vi "Timed_Display.vi"(2 "Message":string, 3 "Seconds to wait":dbl=1.0 format="%.2f") -> (0 "Stopped":bool)   [LabVIEW 2010]
doc: "Waits the number of seconds specified by the Seconds to Wait input, divided by the time dilation factor, if used."
panel:
  in  "stop":bool
  out "Seconds waited":u32(slide) scale=0.0..5.0
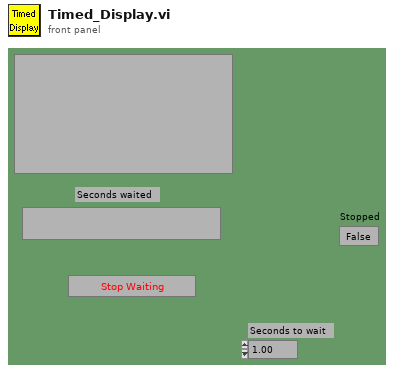
[diagram p1: front panel]
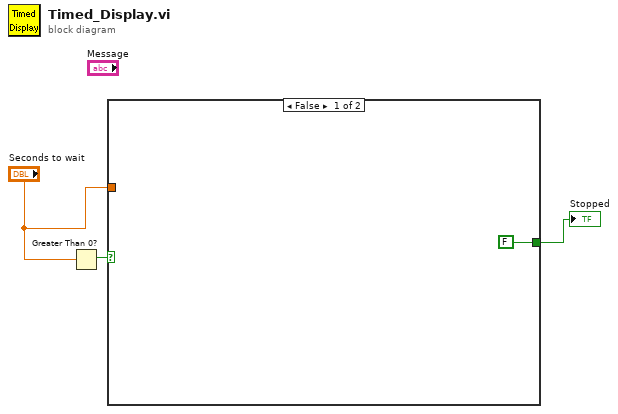
[diagram p0: block diagram]
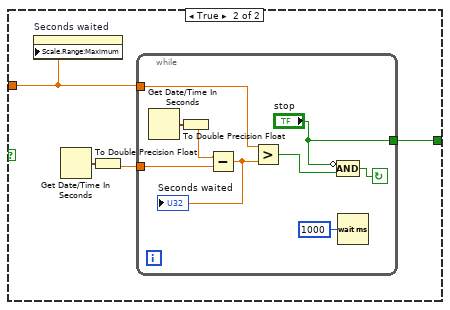
[diagram p2: hidden frame]
diagram:
  n1 = Greater Than 0?(x="Seconds to wait") -> (x > 0?=w3:bool)
  n2 = case shown="False" w3 {
    tunnel: "Seconds to wait" -> [_ w7]
    tunnel: [FALSE ("stop") w5] -> w1
    frame False {
    }
    frame True {
      n3 = property on="Seconds waited" class="Slide (strict)"("Scale.Range:Maximum"=w7) -> ()  [unwired: 2 in, 2 out]
      n4 = Get Date/Time In Seconds() -> (seconds since 1Jan1904=w6:timestamp)
      n5 = To Double Precision Float(number=w6) -> (double precision float=w8:dbl)
      n6 = while {
        tunnel: w7 -> [w16]
        tunnel: w8 -> [w17]
        tunnel: ["stop"] -> w5
        stop <- w10 continue-if-true
        n7 = Get Date/Time In Seconds() -> (seconds since 1Jan1904=w12:timestamp)
        n8 = To Double Precision Float(number=w12) -> (double precision float=w13:dbl)
        n9 = Subtract(x=w13, y=w17) -> (x-y=w15:dbl)
        "Seconds waited" <- w15
        n10 = Greater?(x=w16, y=w15) -> (0:w11:bool)
        n11 = Compound Arithmetic op=AND(invert "stop", w11) -> (w10:bool)
        n12 = Wait (ms)(milliseconds to wait=u32 1000) -> ()  [unwired: 1 out]
      }
    }
  }
  "Stopped" <- w1
